vi "Read RawData.vi"(8 "error in (no error)":errorcluster, 9 "WCM_max_value":bool, 10 "# of scans":i32, 11 "VIS-IR in":refnum<class "VIS-NIR.lvclass">) -> (0 "error out":errorcluster, 1 "Channel II":sgl[][](array[numeric]), 2 "Channel I":sgl[][](array[numeric]), 3 "VIS-IR out":refnum<class "VIS-NIR.lvclass">, 4 "WCM_values":sgl[](array[numeric]))   [LabVIEW 2020, in "VIS-NIR.lvclass"]
uses:
  VIS-NIR.lvclass
  C:/dev/TRANCON/Classes/GeneralFunctionality/GeneralFunctionality.lvclass
  C:/dev/TRANCON/Classes/Detector/Detector.lvclass
  GeneralFunctionality/GeneralFunctionality.lvclass/GeneralFunctionality.ctl
  Detector.lvclass/Detector.ctl
  <vilib>/addons/zeromq/zmq_socket.lvclass
  Detector.lvclass
  GeneralFunctionality/GeneralFunctionality.lvclass
panel:
  out "II CLEAN":i32[](graph)
  out "II RAW":i32[](graph)
  in  "Make visible":bool
  in  "WCM":bool
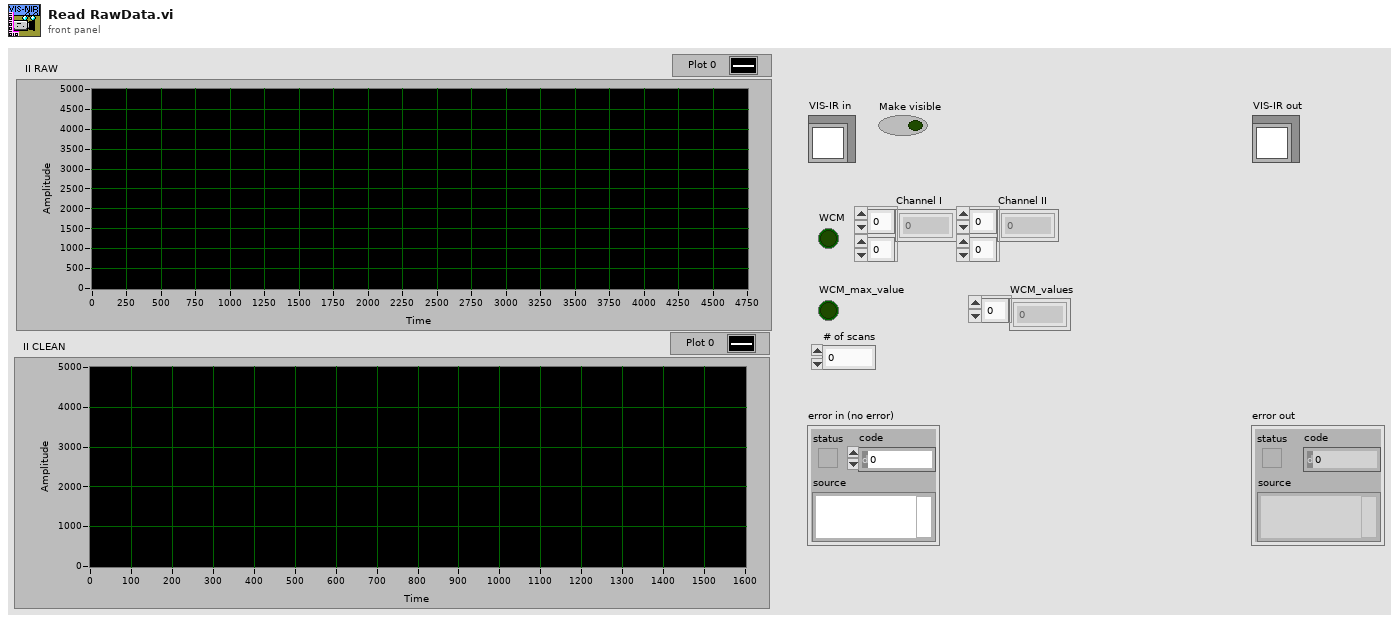
[diagram p1: front panel]
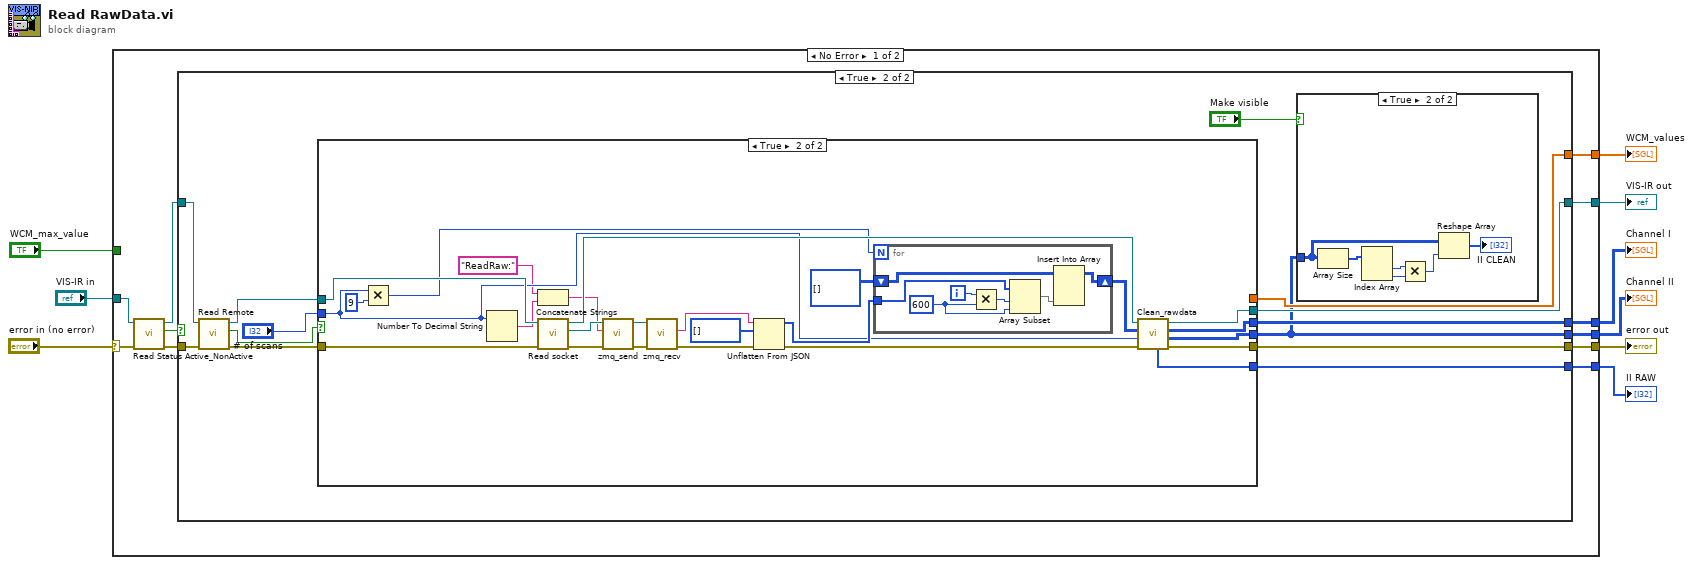
[diagram p0: block diagram]
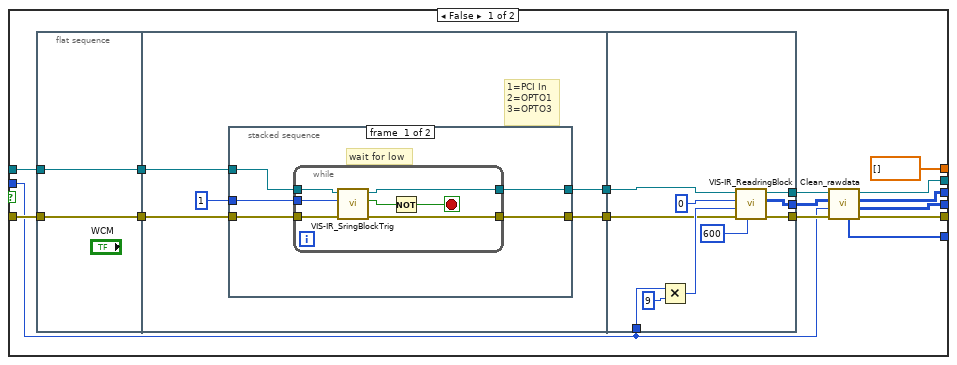
[diagram p4: hidden frame]
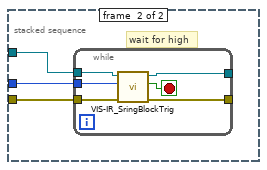
[diagram p5: hidden frame]
diagram:
  n1 = case shown="No Error" "error in (no error)" {
    selector: "error in (no error)" -> [w17 w128]
    tunnel: [w19 w129] -> w8
    tunnel: "VIS-IR in" -> [w14 w129]
    tunnel: [w20 w128] -> w6
    tunnel: "WCM_max_value" -> [_ _]
    tunnel: [w18 _] -> w4
    tunnel: [w12 _] -> w3
    tunnel: [w11 _] -> w2
    tunnel: [w10 _] -> w1
    frame No Error {
      n2 = call "Read Status Active_NonActive.vi"("error in (no error)"=w17, "GeneralFunctionality in"=w14) -> ("error out"=w16:errorcluster, "Status Active/NonActive"=w13:bool, "GeneralFunctionality out"=w15:refnum<class "VIS-NIR.lvclass">)  [unwired: 7 in]
      n3 = case shown="True" w13 {
        tunnel: [w21 w35] -> w20
        tunnel: [w22 w27] -> w19
        tunnel: [_ w34] -> w18
        tunnel: w16 -> [w21 w33]
        tunnel: w15 -> [w22 w32]
        tunnel: [_ w25] -> w12
        tunnel: [_ w24] -> w11
        tunnel: [_ w23] -> w10
        frame False {
        }
        frame True {
          n4 = call "Read Remote.vi"("error in (no error)"=w33, "Detector in"=w32) -> ("error out"=w30:errorcluster, "Remote"=w29:bool, "Detector out"=w31:refnum<class "VIS-NIR.lvclass">)  [unwired: 7 in]
          n5 = case shown="True" w29 {
            tunnel: [w46 w109] -> w35
            tunnel: [dbl[] [] _] -> w34
            tunnel: w31 -> [w52 w119]
            tunnel: w30 -> [w51 w120]
            tunnel: [w44 w107] -> w24
            tunnel: [w45 w108] -> w25
            tunnel: [w43 w106] -> w23
            tunnel: [w47 w110] -> w27
            tunnel: "# of scans" -> [w42 w99]
            frame False {
              n6 = flat-sequence {
                tunnel: [w58] -> w57
                tunnel: [w59] -> w56
                tunnel: w52 -> [w59]
                tunnel: w51 -> [w58]
                tunnel: w57 -> [w62]
                tunnel: w56 -> [w63]
                tunnel: [w61] -> w55
                tunnel: [w60] -> w54
                tunnel: [w92] -> w49
                tunnel: [w95] -> w48
                tunnel: [w94] -> w50
                tunnel: w55 -> [w87]
                tunnel: w54 -> [w88]
                tunnel: w42 -> [w86]
                frame #0 {
                }
                frame #1 {
                  # "1=PCI In\n2=OPTO1\n3=OPTO3"
                  n7 = stacked-sequence {
                    tunnel: u8 1 -> [w69 w79]
                    tunnel: w63 -> [w68 w78]
                    tunnel: w62 -> [w67 w77]
                    tunnel: [w65 _] -> w61
                    tunnel: [w66 _] -> w60
                    frame #0 {
                      # "wait for low"
                      n8 = while {
                        tunnel: w69 -> [w75]
                        tunnel: w68 -> [w74]
                        tunnel: w67 -> [w73]
                        tunnel: [w72] -> w65
                        tunnel: [w71] -> w66
                        stop <- w76 stop-if-true
                        n9 = call "VIS-IR_SringBlockTrig.vi"("error in (no error)"=w73, "channel 1, 2 or 3"=w75, "VIS-IR in"=w74) -> ("error out"=w72:errorcluster, "Boolesch"=w70:bool, "VIS-IR out"=w71:refnum<class "VIS-NIR.lvclass">)  [unwired: 6 in]
                        n10 = Not(x=w70) -> (.not. x?=w76:bool)
                      }
                    }
                    frame #1 {
                      # "wait for high"
                      n11 = while {
                        tunnel: w79 -> [w80]
                        tunnel: w78 -> [w85]
                        tunnel: w77 -> [w84]
                        tunnel: [w83] -> _
                        tunnel: [w82] -> _
                        stop <- w81 stop-if-true
                        n12 = call "VIS-IR_SringBlockTrig.vi"("error in (no error)"=w84, "channel 1, 2 or 3"=w80, "VIS-IR in"=w85) -> ("error out"=w83:errorcluster, "Boolesch"=w81:bool, "VIS-IR out"=w82:refnum<class "VIS-NIR.lvclass">)  [unwired: 6 in]
                      }
                    }
                  }
                }
                frame #2 {
                  n13 = Multiply(x=w86, y=9) -> (x*y=w89:i32)
                  n14 = call "VIS-IR_ReadringBlock.vi"("pixel"=u32 600, "error in (no error)"=w87, "stop"=w89, "start"=0, "VIS-IR in"=w88) -> ("error out"=w92:errorcluster, "Data Values"=w95:u32[][], "VIS-IR out"=w94:refnum<class "VIS-NIR.lvclass">)  [unwired: 4 in]
                }
              }
              n15 = call "Clean_rawdata.vi"("error in (no error)"=w49, "N of scans"=w42, "Data RAW in"=w48, "VIS-NIR en entrée"=w50) -> ("error out"=w46:errorcluster, "I 2"=w44:i32[][], "I"=w45:i32[][], "VIS-NIR en sortie"=w47:refnum<class "VIS-NIR.lvclass">, "II RAW"=w43:i32[])  [unwired: 3 in]
            }
            frame True {
              n16 = Multiply(x=w99, y=9) -> (x*y=w100:i32)
              n17 = Number To Decimal String(number=w99) -> (decimal integer string=w97:string)  [unwired: 1 in]
              n18 = Concatenate Strings("ReadRaw:" ("data"), w97) -> (w96:string)
              n19 = call "Read socket.vi"("error in (no error)"=w120, "Detector in"=w119) -> ("error out"=w118:errorcluster, "zeromq.lvlib:ZeroMQ Socket"=w117:refnum<class "zmq_socket.lvclass">, "Detector out"=w111:refnum<class "VIS-NIR.lvclass">)  [unwired: 7 in]
              n20 = call <vilib>:"zmq_send.vi"("error in"=w118, "data"=w96, "socket in"=w117) -> ("error out"=w116:errorcluster, "socket out"=w115:refnum<class "zmq_socket.lvclass">)  [unwired: 4 in]
              n21 = call <vilib>:"zmq_recv.vi"("error in"=w116, "socket in"=w115) -> ("error out"=w113:errorcluster, "data"=w114:string)  [unwired: 3 in, 3 out]
              n22 = Unflatten From JSON(JSON string=w114, type and defaults=i32[] [] ("array"), error in (no error)=w113) -> (value=w102:i32[], error out=w112:errorcluster)  [unwired: 4 in]
              n23 = for {
                N: w100 -> [_]
                shift-right: [w126] -> w104
                shift-left: i32[][] [] ("array") -> [w127]
                tunnel: w102 -> [w125]
                i -> [w123]
                w121 = 600 ("y")
                n24 = Multiply(x=w123, y=w121) -> (x*y=w122:i32)
                n25 = Array Subset(array=w125, index=w122, length=w121) -> (w124:i32[])
                n26 = Insert Into Array(array=w127, new element=w124) -> (w126:i32[][])  [unwired: 2 in]
              }
              n27 = call "Clean_rawdata.vi"("error in (no error)"=w112, "N of scans"=w99, "Data RAW in"=w104, "VIS-NIR en entrée"=w111) -> ("error out"=w109:errorcluster, "I 2"=w107:i32[][], "I"=w108:i32[][], "VIS-NIR en sortie"=w110:refnum<class "VIS-NIR.lvclass">, "II RAW"=w106:i32[])  [unwired: 3 in]
            }
          }
          n28 = case shown="True" "Make visible" {
            tunnel: w24 -> [_ w37]
            frame False {
            }
            frame True {
              n29 = Array Size(array=w37) -> (size(s)=w38:i32[])
              n30 = Index Array(array=w38) -> (element #1=w39:i32, element #2=w40:i32)  [unwired: 2 in]
              n31 = Multiply(x=w39, y=w40) -> (x*y=w41:i32)
              n32 = Reshape Array(w37, w41) -> (→"II CLEAN":i32[])
            }
          }
        }
      }
    }
    frame Error {
    }
  }
  "error out" <- w6
  "VIS-IR out" <- w8
  "WCM_values" <- w4
  "Channel I" <- w3
  "Channel II" <- w2
  "II RAW" <- w1
